vi "Data_Save_Task_Detect_Calib.vi"(9 "Data":T1) -> (2 "数组":string[](array[string]))   [LabVIEW 2017]
uses:
  Ctrls/Data.ctl
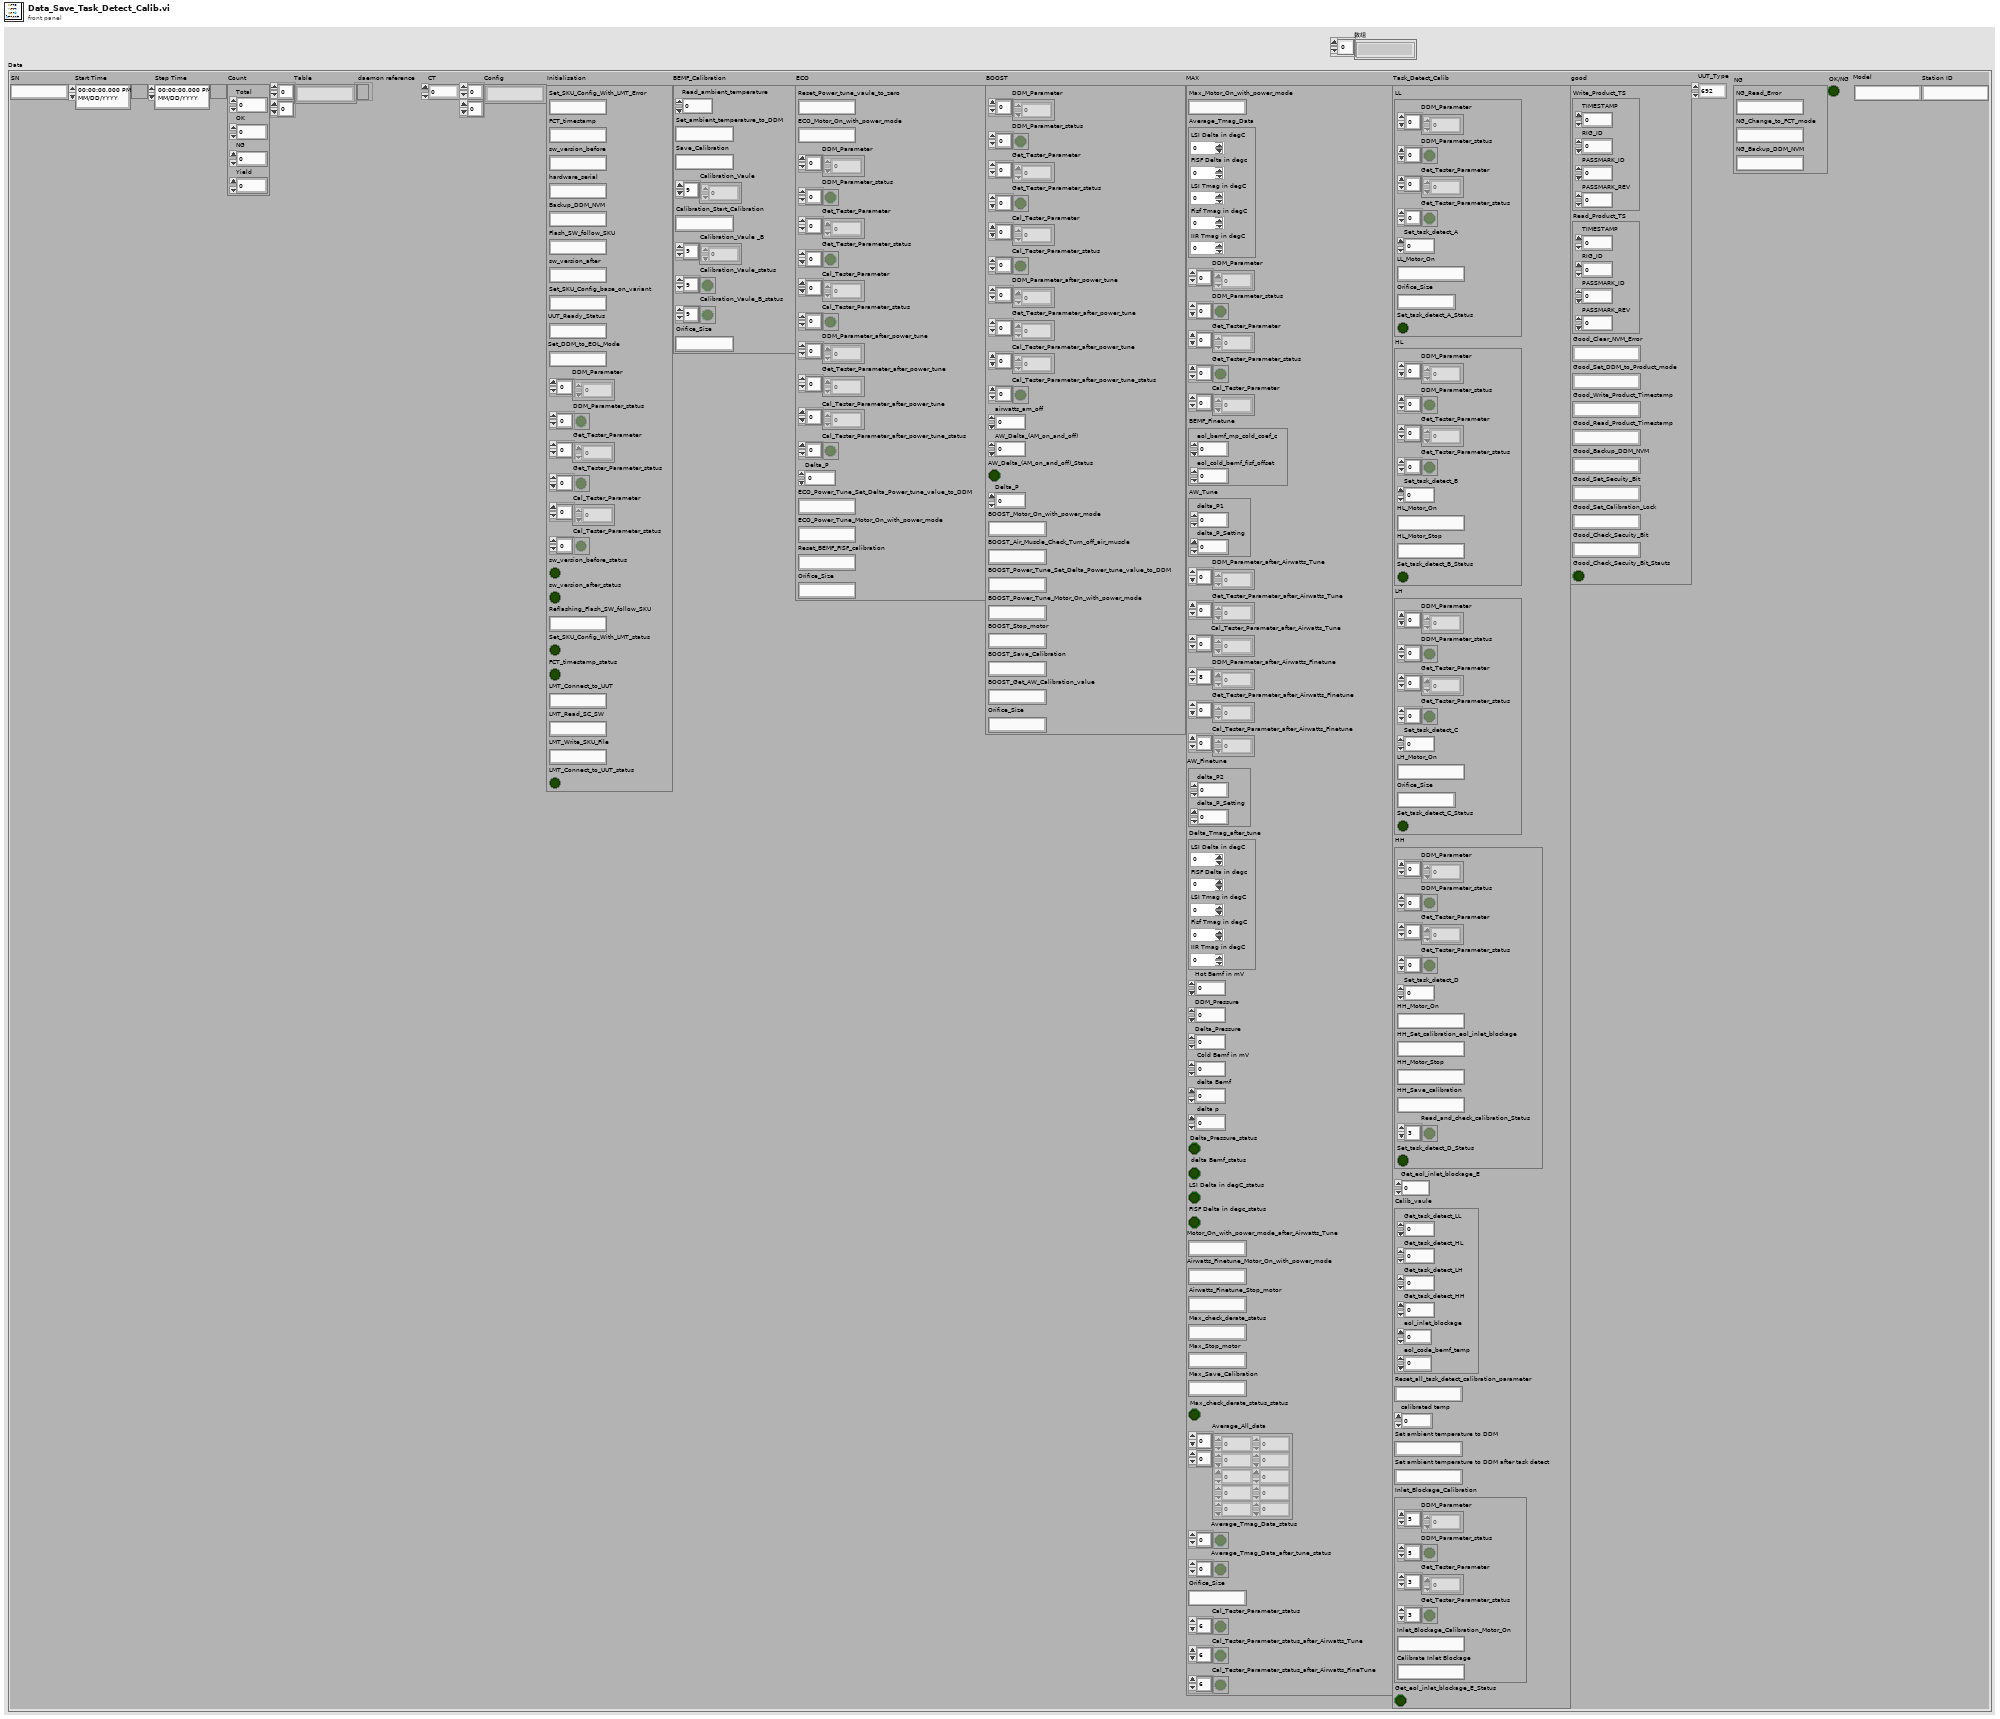
[diagram p1: front panel]
types:
  T1 = typedef "Data.ctl" = cluster{"SN":string, "Start Time":timestamp, "Step Time":timestamp, "Count":cluster{"Total":i32, "OK":i32, "NG":i32, "Yield":dbl}, "Table":string[][], "daemon reference":refnum<k5>, "CT":dbl, "Config":string[][], "Initialisation":cluster{"Set_SKU_Config_With_LMT_Error":string, "FCT_timestamp":string, "sw_version_before":string, "hardware_serial":string, "Backup_DDM_NVM":string, "Flash_SW_follow_SKU":string, "sw_version_after":string, "Set_SKU_Config_base_on_variant":string, "UUT_Ready_Status":string, "Set_DDM_to_EOL_Mode":string, "DDM_Parameter":dbl[], "DDM_Parameter_status":bool[], "Get_Tester_Parameter":dbl[], "Get_Tester_Parameter_status":bool[], "Cal_Tester_Parameter":dbl[], "Cal_Tester_Parameter_status":bool[], "sw_version_before_status":bool, "sw_version_after_status":bool, "Reflashing_Flash_SW_follow_SKU":string, "Set_SKU_Config_With_LMT_status":bool, "FCT_timestamp_status":bool, "LMT_Connect_to_UUT":string, "LMT_Read_SC_SW":string, "LMT_Write_SKU_File":string, "LMT_Connect_to_UUT_status":bool}, "BEMF_Calibration":cluster{"Read_ambient_temperature":dbl, "Set_ambient_temperature_to_DDM":string, "Save_Calibration":string, "Calibration_Vaule":dbl[], "Calibration_Start_Calibration":string, "Calibration_Vaule _B":dbl[], "Calibration_Vaule_status":bool[], "Calibration_Vaule_B_status":bool[], "Orifice_Size":string}, "ECO":cluster{"Reset_Power_tune_vaule_to_zero":string, "ECO_Motor_On_with_power_mode":string, "DDM_Parameter":dbl[], "DDM_Parameter_status":bool[], "Get_Tester_Parameter":dbl[], "Get_Tester_Parameter_status":bool[], "Cal_Tester_Parameter":dbl[], "Cal_Tester_Parameter_status":bool[], "DDM_Parameter_after_power_tune":dbl[], "Get_Tester_Parameter_after_power_tune":dbl[], "Cal_Tester_Parameter_after_power_tune":dbl[], "Cal_Tester_Parameter_after_power_tune_status":bool[], "Delta_P":dbl, "ECO_Power_Tune_Set_Delta_Power_tune_value_to_DDM":string, "ECO_Power_Tune_Motor_On_with_power_mode":string, "Reset_BEMF_FISF_calibration":string, "Orifice_Size":string}, "BOOST":cluster{"DDM_Parameter":dbl[], "DDM_Parameter_status":bool[], "Get_Tester_Parameter":dbl[], "Get_Tester_Parameter_status":bool[], "Cal_Tester_Parameter":dbl[], "Cal_Tester_Parameter_status":bool[], "DDM_Parameter_after_power_tune":dbl[], "Get_Tester_Parameter_after_power_tune":dbl[], "Cal_Tester_Parameter_after_power_tune":dbl[], "Cal_Tester_Parameter_after_power_tune_status":bool[], "airwatts_am_off":dbl, "AW_Delta_(AM_on_and_off)":dbl, "AW_Delta_(AM_on_and_off)_Status":bool, "Delta_P":dbl, "BOOST_Motor_On_with_power_mode":string, "BOOST_Air_Muscle_Check_Turn_off_air_muscle":string, "BOOST_Power_Tune_Set_Delta_Power_tune_value_to_DDM":string, "BOOST_Power_Tune_Motor_On_with_power_mode":string, "BOOST_Stop_motor":string, "BOOST_Save_Calibration":string, "BOOST_Get_AW_Calibration_value":string, "Orifice_Size":string}, "MAX":cluster{"Max_Motor_On_with_power_mode":string, "Average_Tmag_Data":cluster{"LSI Delta in degC":dbl, "FISF Delta in degc":dbl, "LSI Tmag in degC":dbl, "Fisf Tmag in degC":dbl, "IIR Tmag in degC":dbl}, "DDM_Parameter":dbl[], "DDM_Parameter_status":bool[], "Get_Tester_Parameter":dbl[], "Get_Tester_Parameter_status":bool[], "Cal_Tester_Parameter":dbl[], "BEMF_Finetune":cluster{"eol_bemf_mp_cold_coef_c":dbl, "eol_cold_bemf_fisf_offset":dbl}, "AW_Tune":cluster{"delta_P1":dbl, "delta_P_Setting":dbl}, "DDM_Parameter_after_Airwatts_Tune":dbl[], "Get_Tester_Parameter_after_Airwatts_Tune":dbl[], "Cal_Tester_Parameter_after_Airwatts_Tune":dbl[], "DDM_Parameter_after_Airwatts_Finetune":dbl[], "Get_Tester_Parameter_after_Airwatts_Finetune":dbl[], "Cal_Tester_Parameter_after_Airwatts_Finetune":dbl[], "AW_Finetune":cluster{"delta_P2":dbl, "delta_P_Setting":dbl}, "Delta_Tmag_after_tune":cluster{"LSI Delta in degC":dbl, "FISF Delta in degc":dbl, "LSI Tmag in degC":dbl, "Fisf Tmag in degC":dbl, "IIR Tmag in degC":dbl}, "Hot Bemf in mV":dbl, "DDM_Pressure":dbl, "Delta_Pressure":dbl, " Cold Bemf in mV":dbl, " delta Bemf":dbl, " delta p":dbl, "Delta_Pressure_status":bool, " delta Bemf_status":bool, "LSI Delta in degC_status":bool, "FISF Delta in degc_status":bool, "Motor_On_with_power_mode_after_Airwatts_Tune":string, "Airwatts_Finetune_Motor_On_with_power_mode":string, "Airwatts_Finetune_Stop_motor":string, "Max_check_derate_status":string, "Max_Stop_motor":string, "Max_Save_Calibration":string, "Max_check_derate_status_status":bool, "Average_All_data":dbl[][], "Average_Tmag_Data_status":bool[], "Average_Tmag_Data_after_tune_status":bool[], "Orifice_Size":string, "Cal_Tester_Parameter_status":bool[], "Cal_Tester_Parameter_status_after_Airwatts_Tune":bool[], "Cal_Tester_Parameter_status_after_Airwatts_FineTune":bool[]}, "Task_Detect_Calib":cluster{"LL":cluster{"DDM_Parameter":dbl[], "DDM_Parameter_status":bool[], "Get_Tester_Parameter":dbl[], "Get_Tester_Parameter_status":bool[], "Set_task_detect_A":dbl, "LL_Motor_On":string, "Orifice_Size":string, "Set_task_detect_A_Status":bool}, "HL":cluster{"DDM_Parameter":dbl[], "DDM_Parameter_status":bool[], "Get_Tester_Parameter":dbl[], "Get_Tester_Parameter_status":bool[], "Set_task_detect_B":dbl, "HL_Motor_On":string, "HL_Motor_Stop":string, "Set_task_detect_B_Status":bool}, "LH":cluster{"DDM_Parameter":dbl[], "DDM_Parameter_status":bool[], "Get_Tester_Parameter":dbl[], "Get_Tester_Parameter_status":bool[], "Set_task_detect_C":dbl, "LH_Motor_On":string, "Orifice_Size":string, "Set_task_detect_C_Status":bool}, "HH":cluster{"DDM_Parameter":dbl[], "DDM_Parameter_status":bool[], "Get_Tester_Parameter":dbl[], "Get_Tester_Parameter_status":bool[], "Set_task_detect_D":dbl, "HH_Motor_On":string, "HH_Set_calibration_eol_inlet_blockage":string, "HH_Motor_Stop":string, "HH_Save_calibration":string, "Read_and_check_calibration_Status":bool[], "Set_task_detect_D_Status":bool}, "Get_eol_inlet_blockage_E":dbl, "Calib_vaule":cluster{"Get_task_detect_LL":dbl, "Get_task_detect_HL":dbl, "Get_task_detect_LH":dbl, "Get_task_detect_HH":dbl, "eol_inlet_blockage":dbl, "eol_code_bemf_temp":dbl}, "Reset_all_task_detect_calibration_parameter":string, "calibrated temp":dbl, "Set ambient temperature to DDM":string, "Set ambient temperature to DDM after task detect":string, "Inlet_Blockage_Calibration":cluster{"DDM_Parameter":dbl[], "DDM_Parameter_status":bool[], "Get_Tester_Parameter":dbl[], "Get_Tester_Parameter_status":bool[], "Inlet_Blockage_Calibration_Motor_On":string, "Calibrate Inlet Blockage":string}, "Get_eol_inlet_blockage_E_Status":bool}, "good":cluster{"Write_Product_TS":cluster{"TIMESTAMP":i64, "RIG_ID":i64, "PASSMARK_ID":i64, "PASSMARK_REV":i64}, "Read_Product_TS":cluster{"TIMESTAMP":i64, "RIG_ID":i64, "PASSMARK_ID":i64, "PASSMARK_REV":i64}, "Good_Clear_NVM_Error":string, "Good_Set_DDM_to_Product_mode":string, "Good_Write_Product_Timestamp":string, "Good_Read_Product_Timestamp":string, "Good_Backup_DDM_NVM":string, "Good_Set_Secuity_Bit":string, "Good_Set_Calibration_Lock":string, "Good_Check_Secuity_Bit":string, "Good_Check_Secuity_Bit_Stauts":bool}, "UUT_Type":enum16{"692", "692B", "692D"}, "NG":cluster{"NG_Read_Error":string, "NG_Change_to_FCT_mode":string, "NG_Backup_DDM_NVM":string}, "OK/NG":bool, "Model":string, "Station ID":string}
  T2 = cluster{"Get_task_detect_LL":dbl, "Get_task_detect_HL":dbl, "Get_task_detect_LH":dbl, "Get_task_detect_HH":dbl, "eol_inlet_blockage":dbl, "eol_code_bemf_temp":dbl}
  T3 = typedef "HD Config.ctl" = cluster{" PC":cluster{"PC Address":u8[], "PC Port":i32}, "FCO":cluster{"COM":refnum<visa-resource-name>, "Baudrate":u32}, "DC Power ":cluster{"COM":refnum<visa-resource-name>, "Baudrate":u32}, "PW3336":cluster{"COM":refnum<visa-resource-name>, "Baudrate":u32}, "Lefoo":cluster{"COM":refnum<visa-resource-name>, "Baudrate":u32}, "AI Model":cluster{"COM":refnum<visa-resource-name>, "Baudrate":u32}, "DIPC":cluster{"COM":refnum<visa-resource-name>}, "Daemon":cluster{"IP Address":string, "Port":u16, "Retry":u16}, "Motor":cluster{"COM":refnum<visa-resource-name>, "Baudrate":u32}, "G1":bool, "Fail_resume_mode":bool, "Skip DDM Speed&Pressure Passmark":bool}
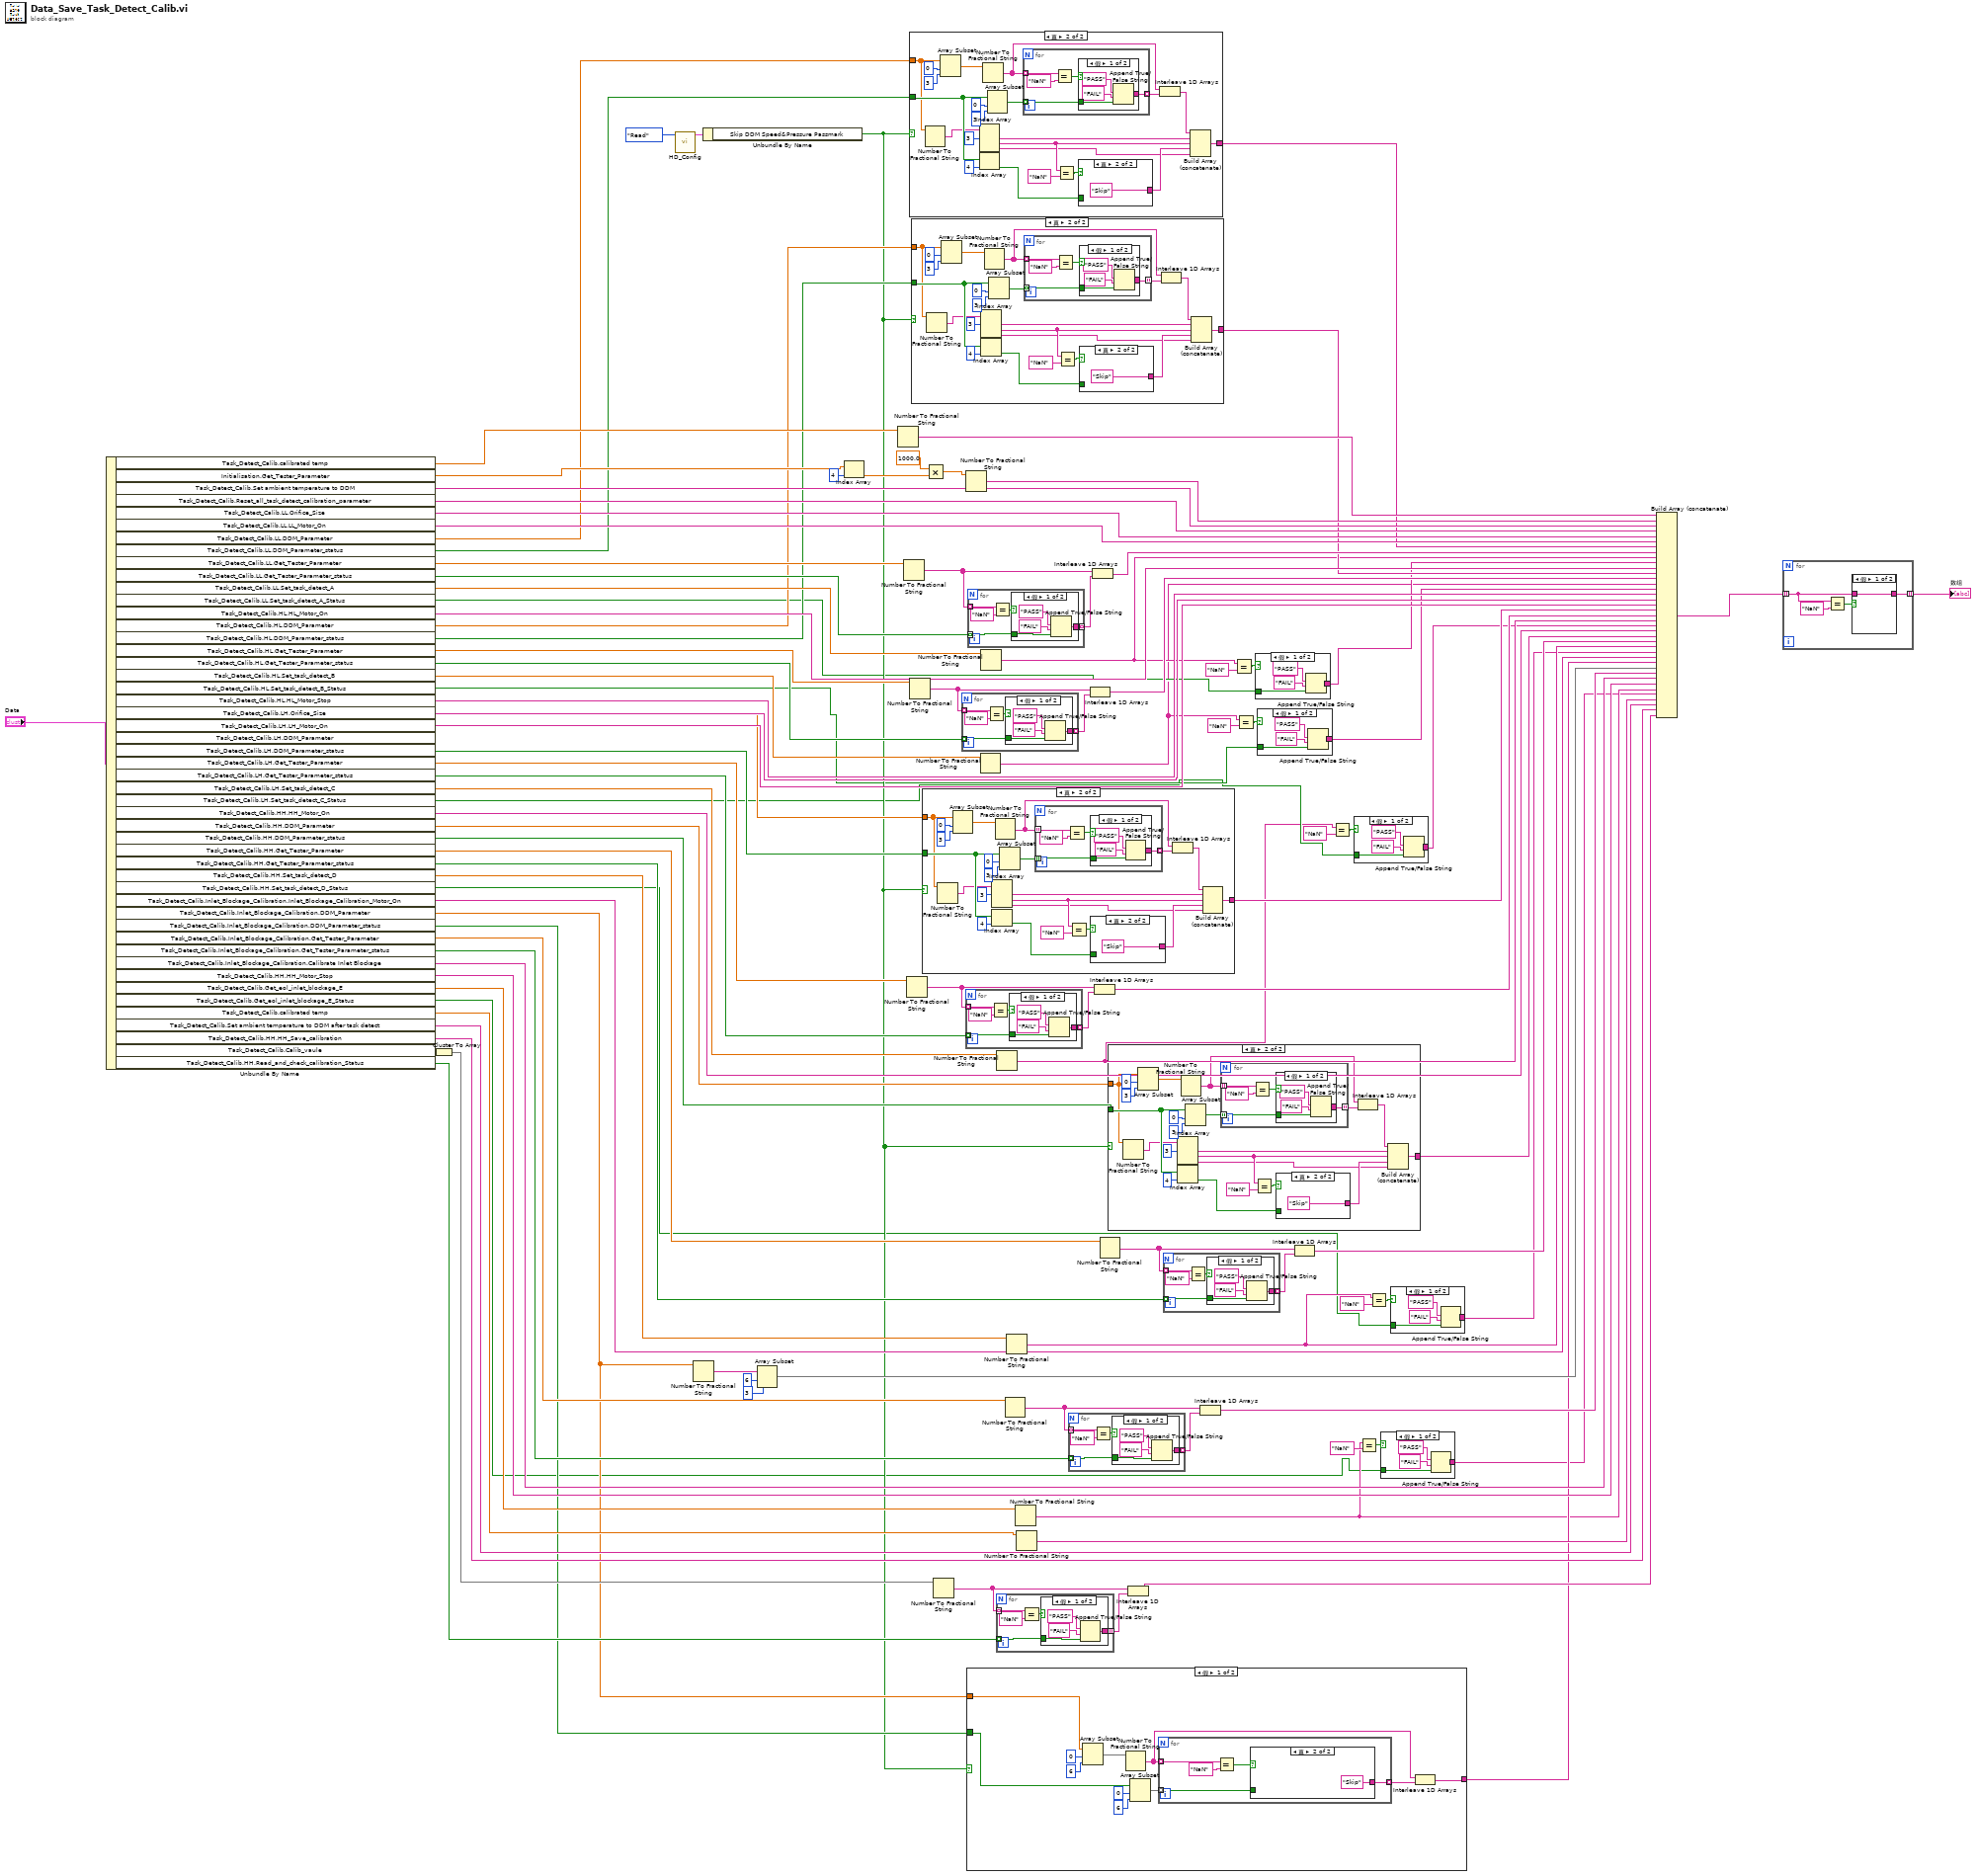
[diagram p0: block diagram]
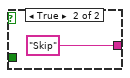
[diagram p2: hidden frame]
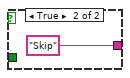
[diagram p3: hidden frame]
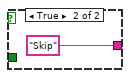
[diagram p4: hidden frame]
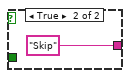
[diagram p5: hidden frame]
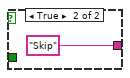
[diagram p6: hidden frame]
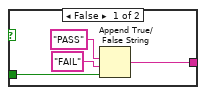
[diagram p7: hidden frame]
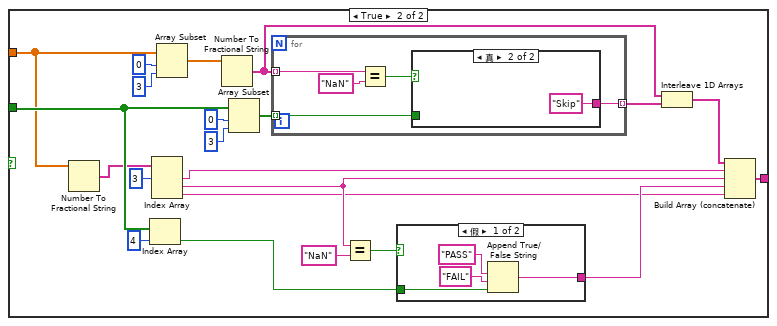
[diagram p8: hidden frame]
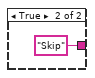
[diagram p9: hidden frame]
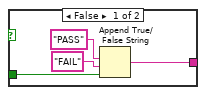
[diagram p10: hidden frame]
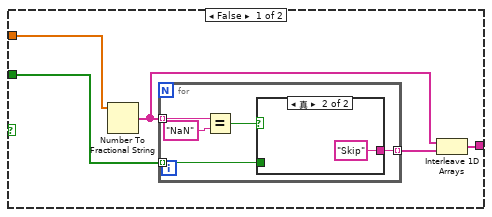
[diagram p11: hidden frame]
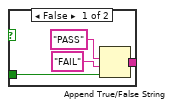
[diagram p12: hidden frame]
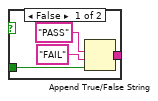
[diagram p13: hidden frame]
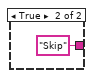
[diagram p14: hidden frame]
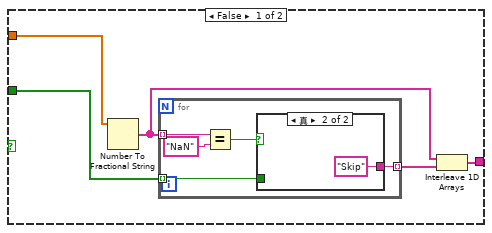
[diagram p15: hidden frame]
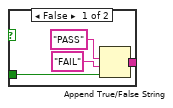
[diagram p16: hidden frame]
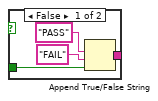
[diagram p17: hidden frame]
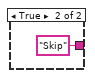
[diagram p18: hidden frame]
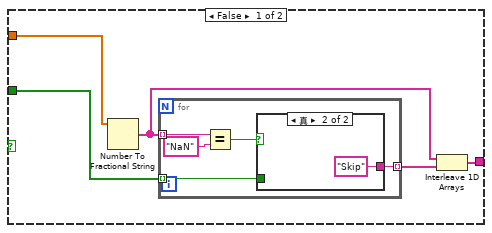
[diagram p19: hidden frame]
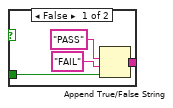
[diagram p20: hidden frame]
diagram:
  n1 = Unbundle By Name("Data") -> ("Task_Detect_Calib.calibrated temp"=w71:dbl, "Initialisation.Get_Tester_Parameter"=w56:dbl[], "Task_Detect_Calib.Set ambient temperature to DDM"=w72:string, "Task_Detect_Calib.Reset_all_task_detect_calibration_parameter"=w73:string, "Task_Detect_Calib.LL.Orifice_Size"=w45:string, "Task_Detect_Calib.LL.LL_Motor_On"=w95:string, "Task_Detect_Calib.LL.DDM_Parameter"=w41:dbl[], "Task_Detect_Calib.LL.DDM_Parameter_status"=w40:bool[], "Task_Detect_Calib.LL.Get_Tester_Parameter"=w109:dbl[], "Task_Detect_Calib.LL.Get_Tester_Parameter_status"=w76:bool[], "Task_Detect_Calib.LL.Set_task_detect_A"=w106:dbl, "Task_Detect_Calib.LL.Set_task_detect_A_Status"=w22:bool, "Task_Detect_Calib.HL.HL_Motor_On"=w94:string, "Task_Detect_Calib.HL.DDM_Parameter"=w38:dbl[], "Task_Detect_Calib.HL.DDM_Parameter_status"=w37:bool[], "Task_Detect_Calib.HL.Get_Tester_Parameter"=w105:dbl[], "Task_Detect_Calib.HL.Get_Tester_Parameter_status"=w79:bool[], "Task_Detect_Calib.HL.Set_task_detect_B"=w104:dbl, "Task_Detect_Calib.HL.Set_task_detect_B_Status"=w17:bool, "Task_Detect_Calib.HL.HL_Motor_Stop"=w93:string, "Task_Detect_Calib.LH.Orifice_Size"=w44:string, "Task_Detect_Calib.LH.LH_Motor_On"=w92:string, "Task_Detect_Calib.LH.DDM_Parameter"=w34:dbl[], "Task_Detect_Calib.LH.DDM_Parameter_status"=w33:bool[], "Task_Detect_Calib.LH.Get_Tester_Parameter"=w102:dbl[], "Task_Detect_Calib.LH.Get_Tester_Parameter_status"=w82:bool[], "Task_Detect_Calib.LH.Set_task_detect_C"=w101:dbl, "Task_Detect_Calib.LH.Set_task_detect_C_Status"=w13:bool, "Task_Detect_Calib.HH.HH_Motor_On"=w91:string, "Task_Detect_Calib.HH.DDM_Parameter"=w32:dbl[], "Task_Detect_Calib.HH.DDM_Parameter_status"=w31:bool[], "Task_Detect_Calib.HH.Get_Tester_Parameter"=w100:dbl[], "Task_Detect_Calib.HH.Get_Tester_Parameter_status"=w84:bool[], "Task_Detect_Calib.HH.Set_task_detect_D"=w99:dbl, "Task_Detect_Calib.HH.Set_task_detect_D_Status"=w7:bool, "Task_Detect_Calib.Inlet_Blockage_Calibration.Inlet_Blockage_Calibration_Motor_On"=w63:string, "Task_Detect_Calib.Inlet_Blockage_Calibration.DDM_Parameter"=w29:dbl[], "Task_Detect_Calib.Inlet_Blockage_Calibration.DDM_Parameter_status"=w28:bool[], "Task_Detect_Calib.Inlet_Blockage_Calibration.Get_Tester_Parameter"=w68:dbl[], "Task_Detect_Calib.Inlet_Blockage_Calibration.Get_Tester_Parameter_status"=w67:bool[], "Task_Detect_Calib.Inlet_Blockage_Calibration.Calibrate Inlet Blockage"=w90:string, "Task_Detect_Calib.HH.HH_Motor_Stop"=w89:string, "Task_Detect_Calib.Get_eol_inlet_blockage_E"=w98:dbl, "Task_Detect_Calib.Get_eol_inlet_blockage_E_Status"=w2:bool, "Task_Detect_Calib.calibrated temp"=w53:dbl, "Task_Detect_Calib.Set ambient temperature to DDM after task detect"=w60:string, "Task_Detect_Calib.HH.HH_Save_calibration"=w88:string, "Task_Detect_Calib.Calib_vaule"=w107:T2, "Task_Detect_Calib.HH.Read_and_check_calibration_Status"=w49:bool[])
  n2 = Cluster To Array(cluster=w107) -> (array=w48:dbl[])
  n3 = call "HD_Config.vi"("Step"=enum16{"Initial", "Write", "Read"}."Read") -> ("HD Config out"=w42:T3)  [unwired: 9 in, 1 out]
  n4 = Number To Fractional String(number=w29) -> (F-format string=w64:string[])  [unwired: 3 in]
  n5 = Unbundle By Name(w42) -> ("Skip DDM Speed&Pressure Passmark"=w26:bool)
  n6 = Array Subset(array=w64, index=6, length=3) -> (w62:string[])
  n7 = Index Array(array=w56, index=4) -> (element=w57:dbl)
  n8 = Number To Fractional String(number=w71) -> (F-format string=w46:string)  [unwired: 3 in]
  n9 = Number To Fractional String(number=w109) -> (F-format string=w75:string[])  [unwired: 3 in]
  n10 = Number To Fractional String(number=w102) -> (F-format string=w80:string[])  [unwired: 3 in]
  n11 = case shown="真" w26 {
    tunnel: w40 -> [w111 w137]
    tunnel: w41 -> [w112 w134]
    tunnel: [w113 w126] -> w39
    frame False {
      n12 = Number To Fractional String(number=w112) -> (F-format string=w114:string[])  [unwired: 3 in]
      n13 = for {
        tunnel: w111 -> [w120] mode=indexing
        tunnel: [w119] -> w115 mode=indexing
        tunnel: w114 -> [w117] mode=indexing
        n14 = Equal?(x=w117, y="NaN" ("x")) -> (x = y?=w116:bool)
        n15 = case shown="真" w116 {
          tunnel: w120 -> [w124 _]
          tunnel: [w122 "Skip" ("x")] -> w119
          frame False {
            n16 = Append True/False String(1:w124, 2:"FAIL" ("字符串(\"\")"), 3:"PASS" ("真字符串")) -> (0:w122:string)  [unwired: 1 in]
          }
          frame True {
          }
        }
      }
      n17 = Interleave 1D Arrays(w114, w115) -> (w113:string[])
    }
    frame True {
      n18 = Number To Fractional String(number=w134) -> (F-format string=w133:string[])  [unwired: 3 in]
      n19 = Array Subset(array=w134, index=0 ("索引"), length=3 ("长度")) -> (w145:dbl[])
      n20 = Index Array(array=w133, index #1=3 ("索引")) -> (element #1=w131:string, element #2=w129:string, element #3=w128:string)  [unwired: 2 in]
      n21 = Index Array(array=w137, index=4 ("索引")) -> (element=w132:bool)
      n22 = Number To Fractional String(number=w145) -> (F-format string=w140:string[])  [unwired: 3 in]
      n23 = Array Subset(array=w137, index=0 ("索引"), length=3 ("长度")) -> (w146:bool[])
      n24 = for {
        tunnel: w146 -> [w157] mode=indexing
        tunnel: [w156] -> w147 mode=indexing
        tunnel: w140 -> [w154] mode=indexing
        n25 = Equal?(x=w154, y="NaN" ("x")) -> (x = y?=w153:bool)
        n26 = case shown="假" w153 {
          tunnel: w157 -> [w161 _]
          tunnel: [w159 "Skip" ("x")] -> w156
          frame False {
            n27 = Append True/False String(1:w161, 2:"FAIL" ("字符串(\"\")"), 3:"PASS" ("真字符串")) -> (0:w159:string)  [unwired: 1 in]
          }
          frame True {
          }
        }
      }
      n28 = Equal?(x=w129, y="NaN" ("x")) -> (x = y?=w136:bool)
      n29 = case shown="真" w136 {
        tunnel: w132 -> [w151 _]
        tunnel: [w149 "Skip" ("x")] -> w130
        frame False {
          n30 = Append True/False String(1:w151, 2:"FAIL" ("字符串(\"\")"), 3:"PASS" ("真字符串")) -> (0:w149:string)  [unwired: 1 in]
        }
        frame True {
        }
      }
      n31 = Interleave 1D Arrays(w140, w147) -> (w127:string[])
      n32 = Build Array (concatenate)(w127, w131, w129, w130, w128) -> (w126:string[])
    }
  }
  n33 = Number To Fractional String(number=w105) -> (F-format string=w77:string[])  [unwired: 3 in]
  n34 = case shown="真" w26 {
    tunnel: w37 -> [w163 w189]
    tunnel: w38 -> [w164 w186]
    tunnel: [w165 w178] -> w36
    frame False {
      n35 = Number To Fractional String(number=w164) -> (F-format string=w166:string[])  [unwired: 3 in]
      n36 = for {
        tunnel: w163 -> [w172] mode=indexing
        tunnel: [w171] -> w167 mode=indexing
        tunnel: w166 -> [w169] mode=indexing
        n37 = Equal?(x=w169, y="NaN" ("x")) -> (x = y?=w168:bool)
        n38 = case shown="真" w168 {
          tunnel: w172 -> [w176 _]
          tunnel: [w174 "Skip" ("x")] -> w171
          frame False {
            n39 = Append True/False String(1:w176, 2:"FAIL" ("字符串(\"\")"), 3:"PASS" ("真字符串")) -> (0:w174:string)  [unwired: 1 in]
          }
          frame True {
          }
        }
      }
      n40 = Interleave 1D Arrays(w166, w167) -> (w165:string[])
    }
    frame True {
      n41 = Number To Fractional String(number=w186) -> (F-format string=w185:string[])  [unwired: 3 in]
      n42 = Array Subset(array=w186, index=0 ("索引"), length=3 ("长度")) -> (w197:dbl[])
      n43 = Index Array(array=w185, index #1=3 ("索引")) -> (element #1=w183:string, element #2=w181:string, element #3=w180:string)  [unwired: 2 in]
      n44 = Index Array(array=w189, index=4 ("索引")) -> (element=w184:bool)
      n45 = Number To Fractional String(number=w197) -> (F-format string=w192:string[])  [unwired: 3 in]
      n46 = Array Subset(array=w189, index=0 ("索引"), length=3 ("长度")) -> (w198:bool[])
      n47 = for {
        tunnel: w198 -> [w209] mode=indexing
        tunnel: [w208] -> w199 mode=indexing
        tunnel: w192 -> [w206] mode=indexing
        n48 = Equal?(x=w206, y="NaN" ("x")) -> (x = y?=w205:bool)
        n49 = case shown="假" w205 {
          tunnel: w209 -> [w213 _]
          tunnel: [w211 "Skip" ("x")] -> w208
          frame False {
            n50 = Append True/False String(1:w213, 2:"FAIL" ("字符串(\"\")"), 3:"PASS" ("真字符串")) -> (0:w211:string)  [unwired: 1 in]
          }
          frame True {
          }
        }
      }
      n51 = Equal?(x=w181, y="NaN" ("x")) -> (x = y?=w188:bool)
      n52 = case shown="真" w188 {
        tunnel: w184 -> [w203 _]
        tunnel: [w201 "Skip" ("x")] -> w182
        frame False {
          n53 = Append True/False String(1:w203, 2:"FAIL" ("字符串(\"\")"), 3:"PASS" ("真字符串")) -> (0:w201:string)  [unwired: 1 in]
        }
        frame True {
        }
      }
      n54 = Interleave 1D Arrays(w192, w199) -> (w179:string[])
      n55 = Build Array (concatenate)(w179, w183, w181, w182, w180) -> (w178:string[])
    }
  }
  n56 = case shown="真" w26 {
    tunnel: w33 -> [w215 w241]
    tunnel: w34 -> [w216 w238]
    tunnel: [w217 w230] -> w35
    frame False {
      n57 = Number To Fractional String(number=w216) -> (F-format string=w218:string[])  [unwired: 3 in]
      n58 = for {
        tunnel: w215 -> [w224] mode=indexing
        tunnel: [w223] -> w219 mode=indexing
        tunnel: w218 -> [w221] mode=indexing
        n59 = Equal?(x=w221, y="NaN" ("x")) -> (x = y?=w220:bool)
        n60 = case shown="真" w220 {
          tunnel: w224 -> [w228 _]
          tunnel: [w226 "Skip" ("x")] -> w223
          frame False {
            n61 = Append True/False String(1:w228, 2:"FAIL" ("字符串(\"\")"), 3:"PASS" ("真字符串")) -> (0:w226:string)  [unwired: 1 in]
          }
          frame True {
          }
        }
      }
      n62 = Interleave 1D Arrays(w218, w219) -> (w217:string[])
    }
    frame True {
      n63 = Number To Fractional String(number=w238) -> (F-format string=w237:string[])  [unwired: 3 in]
      n64 = Array Subset(array=w238, index=0 ("索引"), length=3 ("长度")) -> (w249:dbl[])
      n65 = Index Array(array=w237, index #1=3 ("索引")) -> (element #1=w235:string, element #2=w233:string, element #3=w232:string)  [unwired: 2 in]
      n66 = Index Array(array=w241, index=4 ("索引")) -> (element=w236:bool)
      n67 = Number To Fractional String(number=w249) -> (F-format string=w244:string[])  [unwired: 3 in]
      n68 = Array Subset(array=w241, index=0 ("索引"), length=3 ("长度")) -> (w250:bool[])
      n69 = for {
        tunnel: w250 -> [w261] mode=indexing
        tunnel: [w260] -> w251 mode=indexing
        tunnel: w244 -> [w258] mode=indexing
        n70 = Equal?(x=w258, y="NaN" ("x")) -> (x = y?=w257:bool)
        n71 = case shown="假" w257 {
          tunnel: w261 -> [w265 _]
          tunnel: [w263 "Skip" ("x")] -> w260
          frame False {
            n72 = Append True/False String(1:w265, 2:"FAIL" ("字符串(\"\")"), 3:"PASS" ("真字符串")) -> (0:w263:string)  [unwired: 1 in]
          }
          frame True {
          }
        }
      }
      n73 = Equal?(x=w233, y="NaN" ("x")) -> (x = y?=w240:bool)
      n74 = case shown="真" w240 {
        tunnel: w236 -> [w255 _]
        tunnel: [w253 "Skip" ("x")] -> w234
        frame False {
          n75 = Append True/False String(1:w255, 2:"FAIL" ("字符串(\"\")"), 3:"PASS" ("真字符串")) -> (0:w253:string)  [unwired: 1 in]
        }
        frame True {
        }
      }
      n76 = Interleave 1D Arrays(w244, w251) -> (w231:string[])
      n77 = Build Array (concatenate)(w231, w235, w233, w234, w232) -> (w230:string[])
    }
  }
  n78 = Multiply(x=1000.0, y=w57) -> (x*y=w55:dbl)
  n79 = Number To Fractional String(number=w48) -> (F-format string=w50:string[])  [unwired: 3 in]
  n80 = for {
    tunnel: w79 -> [w271] mode=indexing
    tunnel: [w270] -> w78 mode=indexing
    tunnel: w77 -> [w268] mode=indexing
    n81 = Equal?(x=w268, y="NaN" ("x")) -> (x = y?=w267:bool)
    n82 = case shown="假" w267 {
      tunnel: w271 -> [w275 _]
      tunnel: [w273 "Skip" ("x")] -> w270
      frame False {
        n83 = Append True/False String(1:w275, 2:"FAIL" ("字符串(\"\")"), 3:"PASS" ("真字符串")) -> (0:w273:string)  [unwired: 1 in]
      }
      frame True {
      }
    }
  }
  n84 = Number To Fractional String(number=w55) -> (F-format string=w54:string)  [unwired: 3 in]
  n85 = for {
    tunnel: w82 -> [w281] mode=indexing
    tunnel: [w280] -> w81 mode=indexing
    tunnel: w80 -> [w278] mode=indexing
    n86 = Equal?(x=w278, y="NaN" ("x")) -> (x = y?=w277:bool)
    n87 = case shown="假" w277 {
      tunnel: w281 -> [w285 _]
      tunnel: [w283 "Skip" ("x")] -> w280
      frame False {
        n88 = Append True/False String(1:w285, 2:"FAIL" ("字符串(\"\")"), 3:"PASS" ("真字符串")) -> (0:w283:string)  [unwired: 1 in]
      }
      frame True {
      }
    }
  }
  n89 = case shown="假" w26 {
    tunnel: w28 -> [w288 w319]
    tunnel: w29 -> [w289 w316]
    tunnel: [w287 w308] -> w27
    frame False {
      n90 = Array Subset(array=w289, index=0 ("索引"), length=6 ("长度")) -> (w295:dbl[])
      n91 = Number To Fractional String(number=w295) -> (F-format string=w294:string[])  [unwired: 3 in]
      n92 = Array Subset(array=w288, index=0 ("索引"), length=6 ("长度")) -> (w296:bool[])
      n93 = for {
        tunnel: w296 -> [w302] mode=indexing
        tunnel: [w301] -> w297 mode=indexing
        tunnel: w294 -> [w299] mode=indexing
        n94 = Equal?(x=w299, y="NaN" ("x")) -> (x = y?=w298:bool)
        n95 = case shown="真" w298 {
          tunnel: w302 -> [w306 _]
          tunnel: [w304 "Skip" ("x")] -> w301
          frame False {
            n96 = Append True/False String(1:w306, 2:"FAIL" ("字符串(\"\")"), 3:"PASS" ("真字符串")) -> (0:w304:string)  [unwired: 1 in]
          }
          frame True {
          }
        }
      }
      n97 = Interleave 1D Arrays(w294, w297) -> (w287:string[])
    }
    frame True {
      n98 = Number To Fractional String(number=w316) -> (F-format string=w315:string[])  [unwired: 3 in]
      n99 = Index Array(array=w319, index=4 ("索引")) -> (element=w314:bool)
      n100 = Index Array(array=w315, index #1=3 ("索引")) -> (element #1=w313:string, element #2=w311:string, element #3=w310:string)  [unwired: 2 in]
      n101 = Array Subset(array=w316, index=0 ("索引"), length=3 ("长度")) -> (w327:dbl[])
      n102 = Number To Fractional String(number=w327) -> (F-format string=w322:string[])  [unwired: 3 in]
      n103 = Array Subset(array=w319, index=0 ("索引"), length=3 ("长度")) -> (w328:bool[])
      n104 = for {
        tunnel: w328 -> [w339] mode=indexing
        tunnel: [w338] -> w329 mode=indexing
        tunnel: w322 -> [w336] mode=indexing
        n105 = Equal?(x=w336, y="NaN" ("x")) -> (x = y?=w335:bool)
        n106 = case shown="真" w335 {
          tunnel: w339 -> [w343 _]
          tunnel: [w341 "Skip" ("x")] -> w338
          frame False {
            n107 = Append True/False String(1:w343, 2:"FAIL" ("字符串(\"\")"), 3:"PASS" ("真字符串")) -> (0:w341:string)  [unwired: 1 in]
          }
          frame True {
          }
        }
      }
      n108 = Equal?(x=w311, y="NaN" ("x")) -> (x = y?=w318:bool)
      n109 = case shown="假" w318 {
        tunnel: w314 -> [w333 _]
        tunnel: [w331 "Skip" ("x")] -> w312
        frame False {
          n110 = Append True/False String(1:w333, 2:"FAIL" ("字符串(\"\")"), 3:"PASS" ("真字符串")) -> (0:w331:string)  [unwired: 1 in]
        }
        frame True {
        }
      }
      n111 = Interleave 1D Arrays(w322, w329) -> (w309:string[])
      n112 = Build Array (concatenate)(w309, w313, w311, w312, w310) -> (w308:string[])
    }
  }
  n113 = for {
    tunnel: w76 -> [w349] mode=indexing
    tunnel: [w348] -> w74 mode=indexing
    tunnel: w75 -> [w346] mode=indexing
    n114 = Equal?(x=w346, y="NaN" ("x")) -> (x = y?=w345:bool)
    n115 = case shown="假" w345 {
      tunnel: w349 -> [w353 _]
      tunnel: [w351 "Skip" ("x")] -> w348
      frame False {
        n116 = Append True/False String(1:w353, 2:"FAIL" ("字符串(\"\")"), 3:"PASS" ("真字符串")) -> (0:w351:string)  [unwired: 1 in]
      }
      frame True {
      }
    }
  }
  n117 = Number To Fractional String(number=w104) -> (F-format string=w18:string)  [unwired: 3 in]
  n118 = Number To Fractional String(number=w106) -> (F-format string=w23:string)  [unwired: 3 in]
  n119 = Number To Fractional String(number=w101) -> (F-format string=w12:string)  [unwired: 3 in]
  n120 = for {
    tunnel: w49 -> [w359] mode=indexing
    tunnel: [w358] -> w51 mode=indexing
    tunnel: w50 -> [w356] mode=indexing
    n121 = Equal?(x=w356, y="NaN" ("x")) -> (x = y?=w355:bool)
    n122 = case shown="假" w355 {
      tunnel: w359 -> [w363 _]
      tunnel: [w361 "Skip" ("x")] -> w358
      frame False {
        n123 = Append True/False String(1:w363, 2:"FAIL" ("字符串(\"\")"), 3:"PASS" ("真字符串")) -> (0:w361:string)  [unwired: 1 in]
      }
      frame True {
      }
    }
  }
  n124 = Number To Fractional String(number=w68) -> (F-format string=w70:string[])  [unwired: 3 in]
  n125 = Number To Fractional String(number=w99) -> (F-format string=w8:string)  [unwired: 3 in]
  n126 = Number To Fractional String(number=w98) -> (F-format string=w3:string)  [unwired: 3 in]
  n127 = Number To Fractional String(number=w53) -> (F-format string=w52:string)  [unwired: 3 in]
  n128 = for {
    tunnel: w67 -> [w369] mode=indexing
    tunnel: [w368] -> w69 mode=indexing
    tunnel: w70 -> [w366] mode=indexing
    n129 = Equal?(x=w366, y="NaN" ("x")) -> (x = y?=w365:bool)
    n130 = case shown="假" w365 {
      tunnel: w369 -> [w373 _]
      tunnel: [w371 "Skip" ("x")] -> w368
      frame False {
        n131 = Append True/False String(1:w373, 2:"FAIL" ("字符串(\"\")"), 3:"PASS" ("真字符串")) -> (0:w371:string)  [unwired: 1 in]
      }
      frame True {
      }
    }
  }
  n132 = Interleave 1D Arrays(w77, w78) -> (w103:string[])
  n133 = Interleave 1D Arrays(w75, w74) -> (w108:string[])
  n134 = Interleave 1D Arrays(w80, w81) -> (w97:string[])
  n135 = Number To Fractional String(number=w100) -> (F-format string=w83:string[])  [unwired: 3 in]
  n136 = case shown="真" w26 {
    tunnel: w31 -> [w375 w401]
    tunnel: w32 -> [w376 w398]
    tunnel: [w377 w390] -> w30
    frame False {
      n137 = Number To Fractional String(number=w376) -> (F-format string=w378:string[])  [unwired: 3 in]
      n138 = for {
        tunnel: w375 -> [w384] mode=indexing
        tunnel: [w383] -> w379 mode=indexing
        tunnel: w378 -> [w381] mode=indexing
        n139 = Equal?(x=w381, y="NaN" ("x")) -> (x = y?=w380:bool)
        n140 = case shown="真" w380 {
          tunnel: w384 -> [w388 _]
          tunnel: [w386 "Skip" ("x")] -> w383
          frame False {
            n141 = Append True/False String(1:w388, 2:"FAIL" ("字符串(\"\")"), 3:"PASS" ("真字符串")) -> (0:w386:string)  [unwired: 1 in]
          }
          frame True {
          }
        }
      }
      n142 = Interleave 1D Arrays(w378, w379) -> (w377:string[])
    }
    frame True {
      n143 = Number To Fractional String(number=w398) -> (F-format string=w397:string[])  [unwired: 3 in]
      n144 = Array Subset(array=w398, index=0 ("索引"), length=3 ("长度")) -> (w409:dbl[])
      n145 = Index Array(array=w397, index #1=3 ("索引")) -> (element #1=w395:string, element #2=w393:string, element #3=w392:string)  [unwired: 2 in]
      n146 = Index Array(array=w401, index=4 ("索引")) -> (element=w396:bool)
      n147 = Number To Fractional String(number=w409) -> (F-format string=w404:string[])  [unwired: 3 in]
      n148 = Array Subset(array=w401, index=0 ("索引"), length=3 ("长度")) -> (w410:bool[])
      n149 = for {
        tunnel: w410 -> [w421] mode=indexing
        tunnel: [w420] -> w411 mode=indexing
        tunnel: w404 -> [w418] mode=indexing
        n150 = Equal?(x=w418, y="NaN" ("x")) -> (x = y?=w417:bool)
        n151 = case shown="假" w417 {
          tunnel: w421 -> [w425 _]
          tunnel: [w423 "Skip" ("x")] -> w420
          frame False {
            n152 = Append True/False String(1:w425, 2:"FAIL" ("字符串(\"\")"), 3:"PASS" ("真字符串")) -> (0:w423:string)  [unwired: 1 in]
          }
          frame True {
          }
        }
      }
      n153 = Equal?(x=w393, y="NaN" ("x")) -> (x = y?=w400:bool)
      n154 = case shown="真" w400 {
        tunnel: w396 -> [w415 _]
        tunnel: [w413 "Skip" ("x")] -> w394
        frame False {
          n155 = Append True/False String(1:w415, 2:"FAIL" ("字符串(\"\")"), 3:"PASS" ("真字符串")) -> (0:w413:string)  [unwired: 1 in]
        }
        frame True {
        }
      }
      n156 = Interleave 1D Arrays(w404, w411) -> (w391:string[])
      n157 = Build Array (concatenate)(w391, w395, w393, w394, w392) -> (w390:string[])
    }
  }
  n158 = Interleave 1D Arrays(w50, w51) -> (w47:string[])
  n159 = for {
    tunnel: w84 -> [w431] mode=indexing
    tunnel: [w430] -> w85 mode=indexing
    tunnel: w83 -> [w428] mode=indexing
    n160 = Equal?(x=w428, y="NaN" ("x")) -> (x = y?=w427:bool)
    n161 = case shown="假" w427 {
      tunnel: w431 -> [w435 _]
      tunnel: [w433 "Skip" ("x")] -> w430
      frame False {
        n162 = Append True/False String(1:w435, 2:"FAIL" ("字符串(\"\")"), 3:"PASS" ("真字符串")) -> (0:w433:string)  [unwired: 1 in]
      }
      frame True {
      }
    }
  }
  n163 = Interleave 1D Arrays(w70, w69) -> (w61:string[])
  n164 = Equal?(x=w23, y="NaN" ("x")) -> (x = y?=w24:bool)
  n165 = Equal?(x=w18, y="NaN" ("x")) -> (x = y?=w20:bool)
  n166 = case shown="假" w24 {
    tunnel: w22 -> [w440 _]
    tunnel: [w438 "Skip" ("x")] -> w21
    frame False {
      n167 = Append True/False String(1:w440, 2:"FAIL" ("字符串(\"\")"), 3:"PASS" ("真字符串")) -> (0:w438:string)  [unwired: 1 in]
    }
    frame True {
    }
  }
  n168 = case shown="假" w20 {
    tunnel: w17 -> [w445 _]
    tunnel: [w443 "Skip" ("x")] -> w16
    frame False {
      n169 = Append True/False String(1:w445, 2:"FAIL" ("字符串(\"\")"), 3:"PASS" ("真字符串")) -> (0:w443:string)  [unwired: 1 in]
    }
    frame True {
    }
  }
  n170 = Interleave 1D Arrays(w83, w85) -> (w96:string[])
  n171 = Equal?(x=w12, y="NaN" ("x")) -> (x = y?=w14:bool)
  n172 = case shown="假" w14 {
    tunnel: w13 -> [w450 _]
    tunnel: [w448 "Skip" ("x")] -> w11
    frame False {
      n173 = Append True/False String(1:w450, 2:"FAIL" ("字符串(\"\")"), 3:"PASS" ("真字符串")) -> (0:w448:string)  [unwired: 1 in]
    }
    frame True {
    }
  }
  n174 = Equal?(x=w3, y="NaN" ("x")) -> (x = y?=w4:bool)
  n175 = Equal?(x=w8, y="NaN" ("x")) -> (x = y?=w10:bool)
  n176 = case shown="假" w4 {
    tunnel: w2 -> [w455 _]
    tunnel: [w453 "Skip" ("x")] -> w1
    frame False {
      n177 = Append True/False String(1:w455, 2:"FAIL" ("字符串(\"\")"), 3:"PASS" ("真字符串")) -> (0:w453:string)  [unwired: 1 in]
    }
    frame True {
    }
  }
  n178 = case shown="假" w10 {
    tunnel: w7 -> [w460 _]
    tunnel: [w458 "Skip" ("x")] -> w6
    frame False {
      n179 = Append True/False String(1:w460, 2:"FAIL" ("字符串(\"\")"), 3:"PASS" ("真字符串")) -> (0:w458:string)  [unwired: 1 in]
    }
    frame True {
    }
  }
  n180 = Build Array (concatenate)(w46, w54, w72, w73, w45, w95, w39, w108, w23, w21, w94, w36, w103, w18, w16, w93, w44, w92, w35, w97, w12, w11, w91, w30, w96, w8, w6, w63, w27, w62, w61, w90, w89, w3, w1, w52, w60, w88, w47) -> (w87:string[])
  n181 = for {
    tunnel: [w465] -> w86 mode=indexing
    tunnel: w87 -> [w462] mode=indexing
    n182 = Equal?(x=w462, y="NaN" ("x")) -> (x = y?=w463:bool)
    n183 = case shown="假" w463 {
      tunnel: [w466 "Skip" ("x")] -> w465
      tunnel: w462 -> [w466 _]
      frame False {
      }
      frame True {
      }
    }
  }
  "数组" <- w86
